vi "DQMH_API_Get Module Type Info.vi"() -> (3 "ModuleTypes":string[](array[string]))   [LabVIEW 2016]
uses:
  project/Delacor/DQMH/_DQMH New Module/DQMH New Module.lvlib
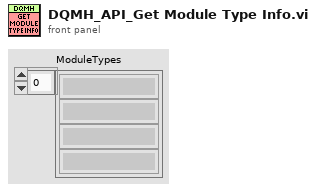
[diagram p1: front panel]
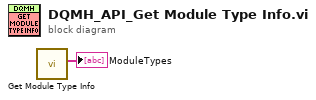
[diagram p0: block diagram]
diagram:
  n1 = call "Get Module Type Info.vi"() -> ("Type Strings"=→"ModuleTypes":string[])  [unwired: 9 in, 2 out]
